vi "BasicControlCall2.vi"(2 "Code":string="Kp=50;\nTi=0.8;\nKflow=2.7e-3;\nu[0]=Kp*(setPoint-h)+u[1];\nif (u[0]<0) u[0] = 0;\nu[1] = u[1] + Kp*dt/Ti * (setPoint - h);\nu[0]=Kflow*u[0];\n", 3 "InitCode":string="u[0]=0;\nu[1]=0;", 4 "plantState":dbl[](array[numeric])=[1.0, 6.74, 0.1], 5 "variablesIN":string="h,setPoint,dt") -> (0 "error":errorcluster, 1 "controlState":dbl[](array[numeric])=[0.7749, 35.875])   [LabVIEW 2013]
panel:
  out "Loaded":bool
  out "error out":errorcluster
  out "restart":bool=TRUE
  in  "variableOUT":string="u"
  out "LastInitCode":string="u[0]=0;\nu[1]=0;"
  in  "Timeout":i32=500
  out "LastCode":string="Kp=50;\nTi=0.8;\nKflow=2.7e-3;\nu[0]=Kp*(setPoint-h)+u[1];\nif (u[0]<0) u[0] = 0;\nu[1] = u[1] + Kp*dt/Ti * (setPoint - h);\nu[0]=Kflow*u[0];\n"
  out "textControlState":string
  out "FullCode":string="function Controller(textPlantState,textControlState)\n{\nvar plantState=textPlantState.split(\",\")\nvar h=Number(plantState[0]);\nvar setPoint=Number(plantState[1]);\nvar dt=Number(plantState[2]);\nvar u=textControlState.split(\",\");\nfor(i = 0; i < u.length; ++i)\n{u[i]=Number(u[i]);}\nKp=50;\nTi=0.8;\nKflow=2.7e-3;\nu[0]=Kp*(setPoint-h)+u[1];\nif (u[0]<0) u[0] = 0;\nu[1] = u[1] + Kp*dt/Ti * (setPoint - h);\nu[0]=Kflow*u[0];\n\nreturn u.toString();\n}\n\nfunction Init(textPlantState,textControlState)\n{\nvar plantState=textPlantState.split(\",\")\nvar h=Number(plantState[0]);\nvar setPoint=Number(plantState[1]);\nvar dt=Number(plantState[2]);\nvar u=textControlState.split(\",\");\nfor(i = 0; i < u.length; ++i)\n{u[i]=Number(u[i]);}\nu[0]=0;\nu[1]=0;\nreturn u.toString();\n}\n"
  out "textPlantState":string="1.000000E+0,6.740000E+0,1.000000E-1"
  in  "ScriptControl":refnum<k7>(container)
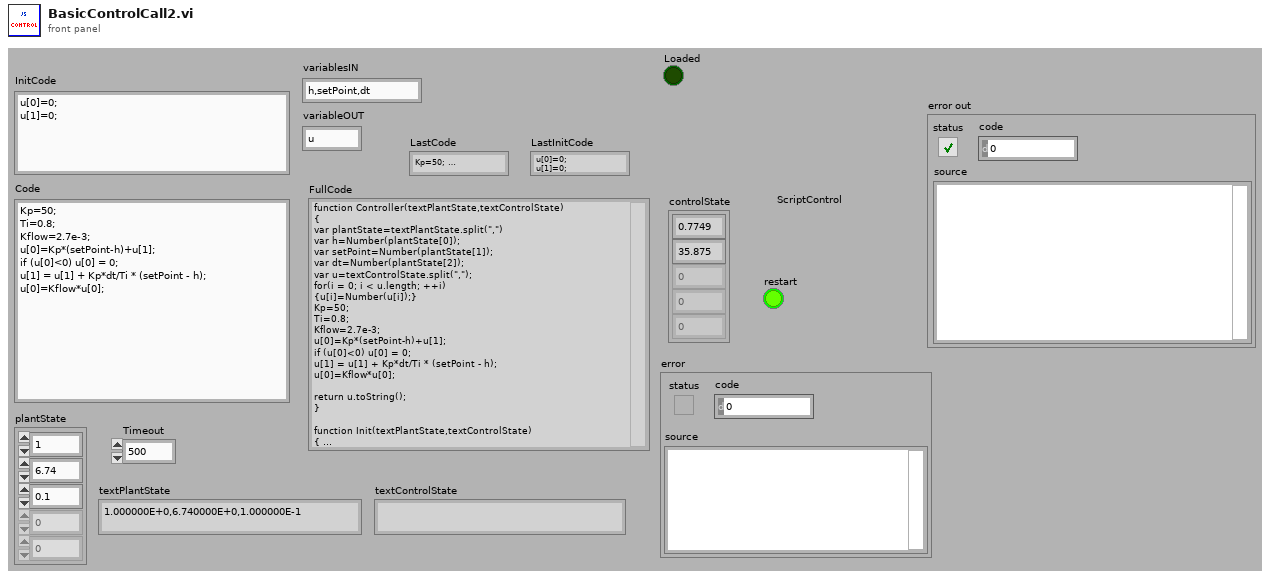
[diagram p1: front panel]
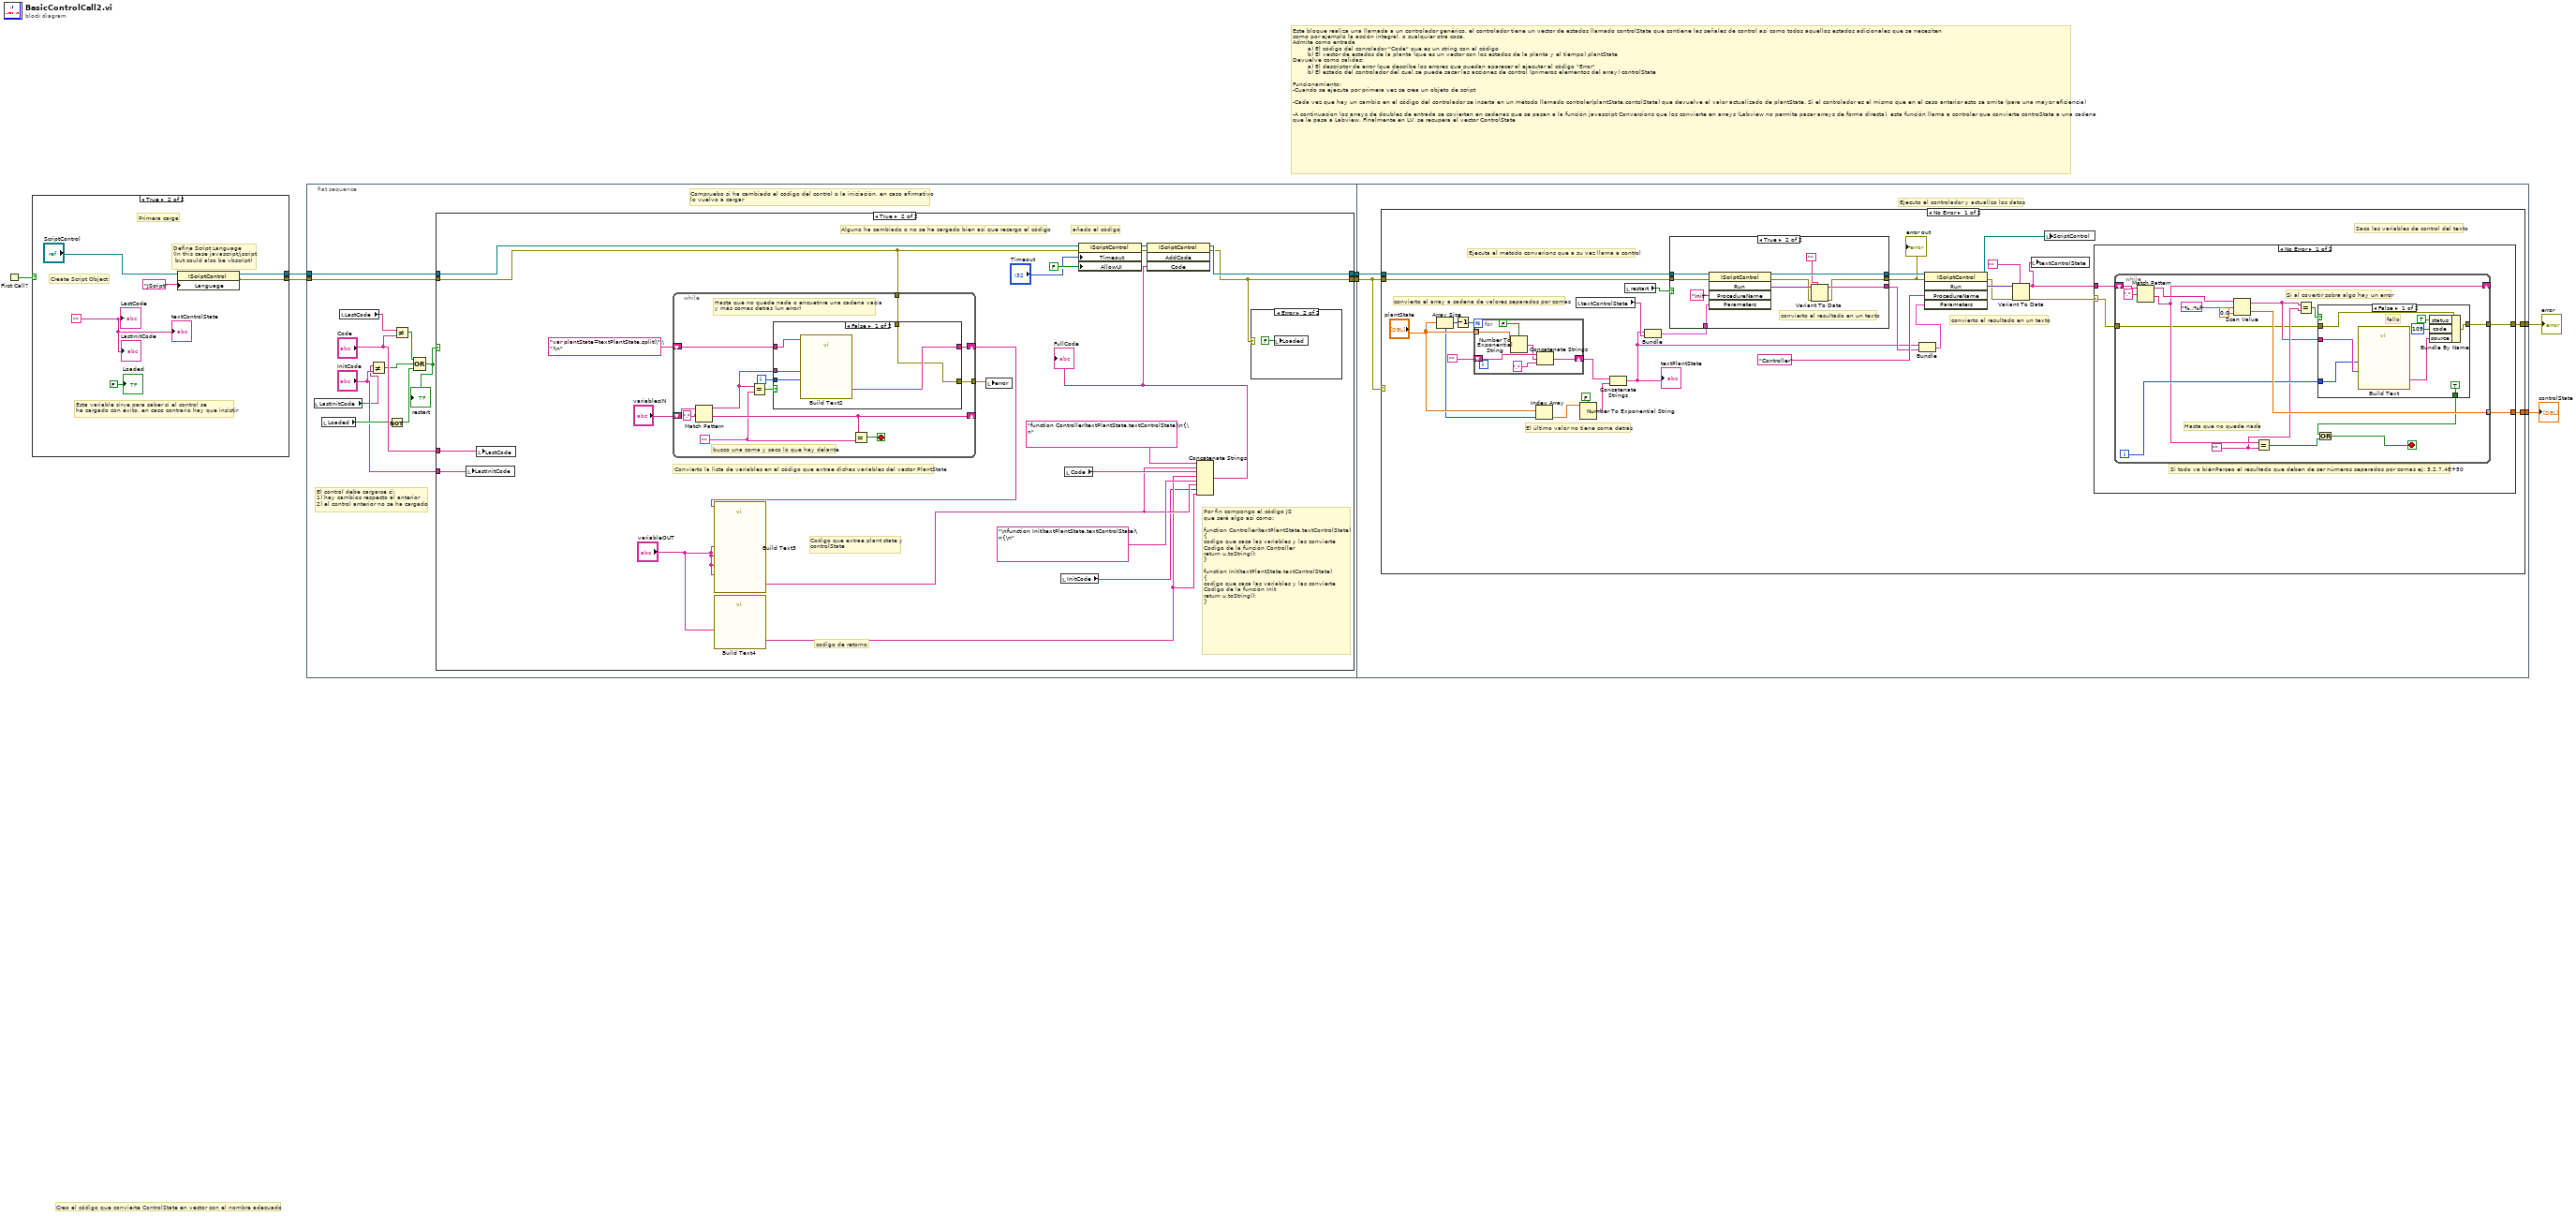
[diagram p0: block diagram]
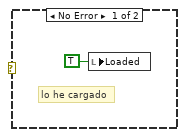
[diagram p3: hidden frame]
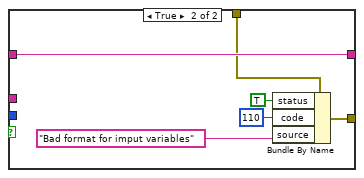
[diagram p4: hidden frame]
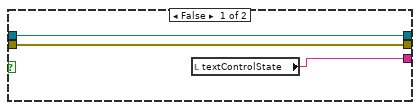
[diagram p5: hidden frame]
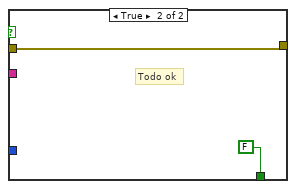
[diagram p6: hidden frame]
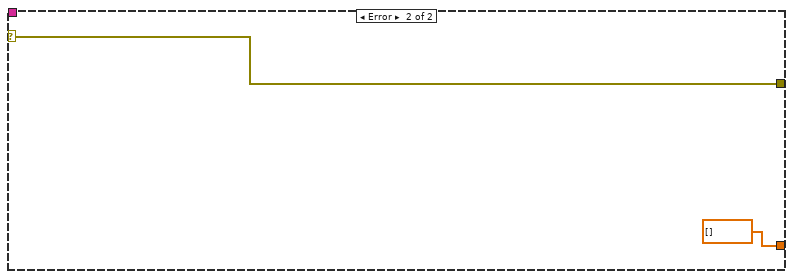
[diagram p7: hidden frame]
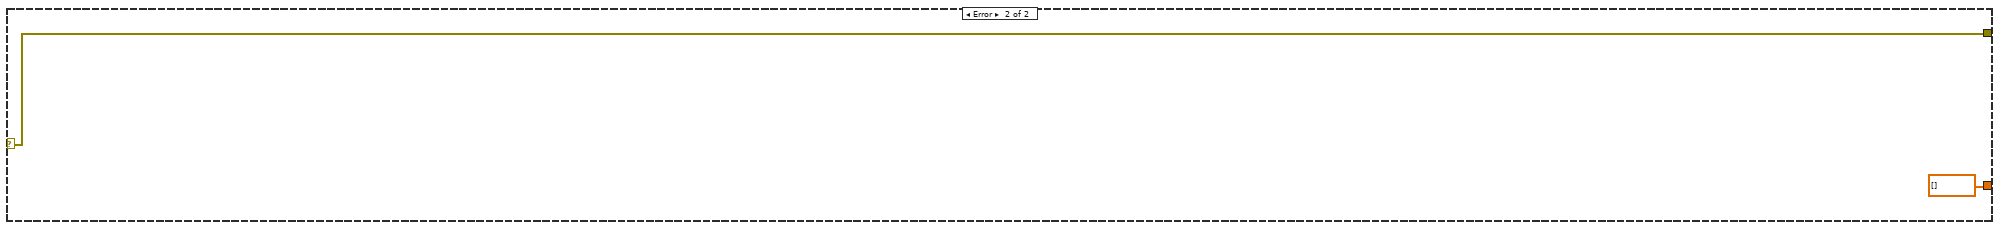
[diagram p8: hidden frame]
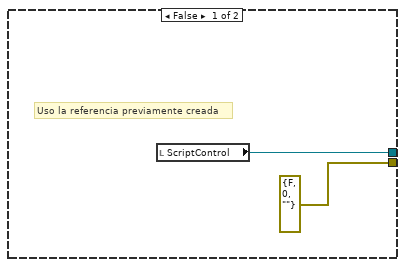
[diagram p9: hidden frame]
diagram:
  # "Creo el código que convierte ControlState en vector con el nombre adecuado"
  # "Este bloque realiza una llamada a un controlador genérico, el controlador tiene un vector de estados llamado controlState que contiene las señales de control así como todos aquellos estados adicionales que se necesiten\ncomo por ejemplo la acción integral, o cualquier otra cosa.\nAdmite como entrada \n        a) El código del conrolador \"Code\" que es un string con el código \n        b) El vector de estados de la planta (que es un vector con los estados de la planta y el tiempo) plantState\nDevuelve como salidas:\n        a) El descriptor de error (que describe los errores que puedan aparecer al ejecutar el código \"Error\"\n        b) El estado del controlador del cual se puede sacar las acciones de control (primeros elementos del array) controlState\n\nFuncionamiento:\n-Cuando se ejecuta por primera vez se crea un objeto de script\n\n-Cada vez que hay un cambio en el código del controlador se inserta en un método llamado controler(plantState,contolState) que devuelve el valor actualizado de plantState. Si el controlador es el mismo que en el caso anterior esto se omite (para una mayor eficiencia)\n \n-A continuacion los arrays de doubles de entrada se covierten en cadenas que se pasan a la función javascript Conversions que los convierte en arrays (Labview no permite pasar arrays de forma directa), esta función llama a controler que convierte controState a una cadena\nque le pasa a Labview. Finalmente en LV, se recupera el vector ControlState"
  n1 = First Call?() -> (First Call?: T/F=w7:bool)
  n2 = case shown="True" w7 {
    tunnel: [w9 w13] -> w6
    tunnel: [errorcluster {"status"=FALSE, "code"=0, "source"=""} ("error out") w12] -> w2
    frame False {
      # "Uso la referencia previamente creada"
      n3 = local read "ScriptControl"() -> (w9:refnum<k7>)
    }
    frame True {
      w11 = ""
      # "Esta variable sirve para saber si el control se \nha cargado con éxito, en caso contrario hay que insistir"
      # "Create Script Object"
      # "Define Script Language\n(In this case javascript/jscript\n but could also be vbscript)"
      # "Primera carga"
      n4 = property class="IScriptControl"(reference="ScriptControl", "Language"="JScript") -> (reference out=w13:refnum<k7>, error out=w12:errorcluster)  [unwired: 1 in]
      "LastCode" <- w11
      "textControlState" <- w11
      "LastInitCode" <- w11
      "Loaded" <- FALSE
    }
  }
  n5 = flat-sequence {
    tunnel: w6 -> [w26]
    tunnel: [w27] -> w5
    tunnel: w2 -> [w25]
    tunnel: [w24] -> w1
    tunnel: w5 -> [w79]
    tunnel: [w81] -> w4
    tunnel: [w80] -> w3
    tunnel: w1 -> [w78]
    frame #0 {
      # "El control debe cargarse si:\n1) hay cambios respecto al anterior\n2) el control anterior no se ha cargado"
      # "Compruebo si ha cambiado el codigo del control o la iniciación, en caso afirmativo\nlo vuelvo a cargar"
      n6 = local read "LastInitCode"() -> (w20:string)
      n7 = local read "Loaded"() -> (w22:bool)
      n8 = local read "LastCode"() -> (w28:string)
      n9 = Not Equal?(x=w20, y="InitCode") -> (x != y?=w18:bool)
      n10 = Not(x=w22) -> (.not. x?=w17:bool)
      n11 = Not Equal?(x=w28, y="Code") -> (x != y?=w19:bool)
      n12 = Compound Arithmetic op=OR(w19, w18, w17) -> (w16:bool)
      "restart" <- w16
      n13 = case shown="True" w16 {
        tunnel: [w30 w52] -> w27
        tunnel: w26 -> [w30 w49]
        tunnel: "Code" -> [_ w36]
        tunnel: w25 -> [w29 w38]
        tunnel: [w29 w31] -> w24
        tunnel: "InitCode" -> [_ w35]
        frame False {
          # "Ambos están cargados y permanecen igual y no hago nada"
        }
        frame True {
          # "codigo de retorno"
          # "Codigo que extrae plant state y\ncontrolState"
          # "Por fin compongo el código JS\nque será algo así como:\n\nfunction Controller(textPlantState,textControlState)\n{\ncodigo que saca las variables y las convierte\nCodigo de la función Controller\nreturn u.toString();\n}\n\nfunction Init(textPlantState,textControlState)\n{\ncodigo que saca las variables y las convierte\nCodigo de la función Init\nreturn u.toString();\n}"
          # "Convierto la lista de variables en el código que extrae dichas variables del vector PlantState"
          # "Alguno ha cambiado o no se ha cargado bien así que recargo el código"
          # "añado el código"
          n14 = local write "LastInitCode"(w35) -> ()
          n15 = local write "LastCode"(w36) -> ()
          n16 = while {
            shift-right: [w64] -> _
            shift-left: "variablesIN" -> [w65]
            shift-right: [w60] -> w43
            shift-left: "var plantState=textPlantState.split(\",\")\n" ("Result") -> [w59]
            tunnel: [w62] -> w40
            tunnel: w38 -> [w55]
            i -> [w57]
            stop <- w63 stop-if-true
            w61 = ""
            # "busco una coma y saco lo que hay delante"
            # "Hasta que no quede nada o encuetnre una cadena vacía\ny más comas detras (un error)"
            n17 = Match Pattern(string=w65, regular expression=",") -> (before substring=w56:string, after substring=w64:string)  [unwired: 1 in, 2 out]
            n18 = Equal?(x=w56, y=w61) -> (x = y?=w58:bool)
            n19 = case shown="False" w58 {
              tunnel: [w67 w74] -> w62
              tunnel: [w71 w73] -> w60
              tunnel: w59 -> [w70 w73]
              tunnel: w57 -> [w69 _]
              tunnel: w56 -> [w68 _]
              tunnel: w55 -> [w67 w72]
              frame False {
                n20 = call "Build Text2"("Beginning Text"=w70, "nombre"=w68, "i"=w69) -> ("Result"=w71:string)  [unwired: 11 in, 1 out]
              }
              frame True {
                n21 = Bundle By Name(cluster=w72, "status"=TRUE, "code"=110, "source"="Bad format for imput variables") -> (w74:errorcluster)
              }
            }
            n22 = Equal?(x=w64, y=w61) -> (x = y?=w63:bool)
          }
          n23 = call "Build Text3"("Beginning Text"=w43, "Uname"="variableOUT", "Uname1"="variableOUT", "Uname2"="variableOUT", "Uname3"="variableOUT") -> ("Result"=w34:string)  [unwired: 9 in, 1 out]
          n24 = call "Build Text4"("Uname"="variableOUT") -> ("Result"=w33:string)  [unwired: 13 in, 1 out]
          n25 = local write "error"(w40) -> ()
          n26 = local read "InitCode"() -> (w32:string)
          n27 = local read "Code"() -> (w45:string)
          n28 = property class="IScriptControl"(reference=w49, error in=w38, "Timeout"="Timeout", "AllowUI"=FALSE) -> (reference out=w50:refnum<k7>, error out=w48:errorcluster)
          n29 = Concatenate Strings("function Controller(textPlantState,textControlState)\n{\n" ("string"), w34, w45, w33, "\nfunction Init(textPlantState,textControlState)\n{\n" ("string"), w34, w32, w33) -> (w37:string)
          "FullCode" <- w37
          n30 = invoke class="IScriptControl" method="AddCode"(reference=w50, error in=w48, "Code"=w37) -> (reference out=w52:refnum<k7>, error out=w31:errorcluster)  [unwired: 1 in, 2 out]
          n31 = case shown="Error" w31 {
            frame No Error {
              # "lo he cargado"
              n32 = local write "Loaded"(TRUE ("Loaded")) -> ()
            }
            frame Error {
              n33 = local write "Loaded"(FALSE ("Loaded")) -> ()
            }
          }
        }
      }
    }
    frame #1 {
      # "Ejecuto el controlador y actualizo los datos"
      n34 = case shown="No Error" w78 {
        selector: w78 -> [_ w161]
        tunnel: [w95 w161] -> w81
        tunnel: [w94 dbl[] [] ("Array")] -> w80
        tunnel: w79 -> [w91 _]
        tunnel: w78 -> [w88 _]
        frame No Error {
          # "Saco las variables de control del texto"
          # "convierto el resultado en un texto"
          # "El último valor no tiene coma detrás"
          # "convierto el array a cadena de valores separados por comas"
          # "Ejecuta el método converions que a su vez llama a control"
          n35 = Array Size(array="plantState") -> (size(s)=w104:i32)
          n36 = Decrement(x=w104) -> (x-1=w105:i32)
          n37 = for {
            N: w105 -> [_]
            tunnel: "plantState" -> [w159] mode=indexing
            shift-right: [w157] -> w99
            shift-left: "" -> [w155]
            n38 = Number To Exponential String(number=w159, 1:FALSE ("use system decimal point (T)")) -> (E-format string=w154:string)  [unwired: 2 in]
            n39 = Concatenate Strings(w155, w154, "," ("string")) -> (w157:string)
          }
          n40 = Index Array(array="plantState", index=w105) -> (element=w102:dbl)
          n41 = local read "textControlState"() -> (w100:string)
          n42 = Number To Exponential String(number=w102, 1:FALSE ("use system decimal point (T)")) -> (E-format string=w103:string)  [unwired: 2 in]
          n43 = Concatenate Strings(w99, w103) -> (w84:string)
          "textPlantState" <- w84
          n44 = local read "restart"() -> (w86:bool)
          n45 = Bundle(w84, "textControlState"=w100) -> (w83:cluster{string, "textControlState":string})  [unwired: 1 in]
          n46 = case shown="True" w86 {
            tunnel: w91 -> [w111 w121]
            tunnel: [w111 w120] -> w90
            tunnel: w88 -> [w110 w119]
            tunnel: [w110 w112] -> w87
            tunnel: w83 -> [_ w118]
            tunnel: [w109 w114] -> w85
            frame False {
              n47 = local read "textControlState"() -> (w109:string)
            }
            frame True {
              # "convierto el resultado en un texto"
              n48 = invoke class="IScriptControl" method="Run"(reference=w121, error in=w119, "ProcedureName"="Init", "Parameters"=w118) -> (reference out=w120:refnum<k7>, error out=w113:errorcluster, "Run"=w116:variant)  [unwired: 1 in, 2 out]
              n49 = Variant To Data(error in=w113, type="", Variant=w116) -> (data=w114:string, error out=w112:errorcluster)
            }
          }
          "error out" <- w87
          n50 = Bundle(w84, "textControlState"=w85) -> (w82:cluster{string, "textControlState":string})  [unwired: 1 in]
          n51 = invoke class="IScriptControl" method="Run"(reference=w90, error in=w87, "ProcedureName"="Controller", "Parameters"=w82) -> (reference out=w92:refnum<k7>, error out=w96:errorcluster, "Run"=w97:variant)  [unwired: 1 in, 2 out]
          n52 = Variant To Data(error in=w96, type="", Variant=w97) -> (data=w93:string, error out=w108:errorcluster)
          n53 = local write "textControlState"(w93) -> ()
          n54 = local write "ScriptControl"(w92) -> ()
          n55 = case shown="No Error" w108 {
            selector: w108 -> [w122 w153]
            tunnel: [w125 dbl[] [] ("Array")] -> w94
            tunnel: w93 -> [w124 _]
            tunnel: [w123 w153] -> w95
            frame No Error {
              # "Si todo va biénParseo el resultado que deben de ser números separados por comas ej: 3.2,7,4E+50"
              n56 = while {
                shift-right: [w130] -> _
                shift-left: w124 -> [w140]
                tunnel: [w138] -> w125 mode=indexing
                tunnel: [w132] -> w123
                tunnel: w122 -> [w126]
                i -> [w135]
                stop <- w133 stop-if-true
                w129 = ""
                # "Hasta que no quede nada"
                # "Si al covertir sobra algo hay un error"
                n57 = Match Pattern(string=w140, regular expression=",") -> (before substring=w131:string, after substring=w130:string)  [unwired: 1 in, 2 out]
                n58 = Scan Value(string=w131, format string="%.;%f", default (0 dbl)=0.0) -> (output string=w128:string, value=w138:dbl)
                n59 = Equal?(x=w130, y=w129) -> (x = y?=w134:bool)
                n60 = Equal?(x=w128, y=w129) -> (x = y?=w127:bool)
                n61 = case shown="False" w127 {
                  tunnel: [TRUE ("x = y?") FALSE ("x = y?")] -> w136
                  tunnel: w135 -> [w143 _]
                  tunnel: w128 -> [w149 _]
                  tunnel: [w147 w150] -> w132
                  tunnel: w126 -> [w142 w150]
                  frame False {
                    # "fallo"
                    n62 = call "Build Text"("num"=w143, "texto"=w149) -> ("Result"=w146:string)  [unwired: 12 in, 1 out]
                    n63 = Bundle By Name(cluster=w142, "status"=TRUE, "code"=109, "source"=w146) -> (w147:errorcluster)
                  }
                  frame True {
                    # "Todo ok"
                  }
                }
                n64 = Or(x=w136, y=w134) -> (x .or. y?=w133:bool)
              }
            }
            frame Error {
            }
          }
        }
        frame Error {
        }
      }
    }
  }
  "error" <- w4
  "controlState" <- w3
